vi "G4BaseTemplate_Singleton_4x4x4_ReadWriteAttribute.vi"(8 "error in (no error)":errorcluster) -> (0 "error out":errorcluster)   [LabVIEW 2016]
uses:
  <resource>/Framework/Providers/Open_GDS/ClassProviders/Provider_EndevoGOOP400/Templates/G4BaseTemplate_Singleton_4x4x4/G4BaseTemplate_Singleton_4x4x4.lvclass
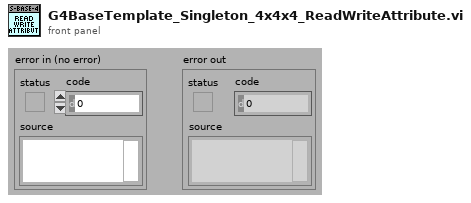
[diagram p1: front panel]
types:
  T1 = typedef "G4BaseTemplate_Singleton_4x4x4.lvclass/ObjectAttributes.ctl" = cluster{"Attribute1":dbl}
  T2 = typedef "G4BaseTemplate_Simple_4x4x4.lvclass/ObjectAttributes.ctl" = cluster{"Attribute1":dbl}
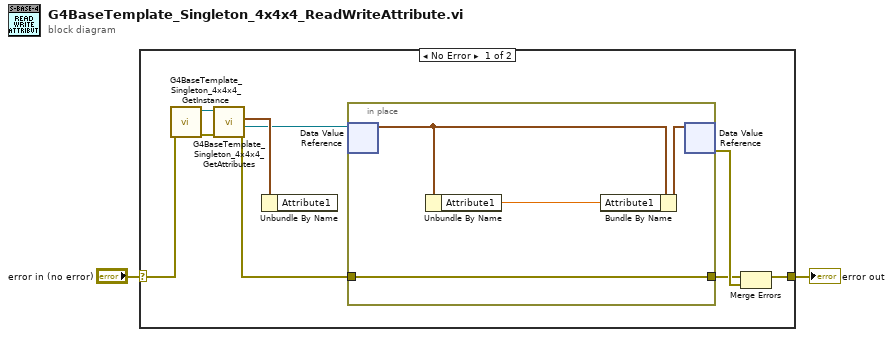
[diagram p0: block diagram]
diagram:
  n1 = case shown="No Error" "error in (no error)" {
    selector: "error in (no error)" -> [w6 w16]
    tunnel: [w9 w16] -> w1
    frame No Error {
      n2 = call <resource>:"G4BaseTemplate_Singleton_4x4x4_GetInstance.vi"("error in (no error)"=w6) -> ("error out"=w8:errorcluster, "reference out"=w7:refnum<class "G4BaseTemplate_Singleton_4x4x4.lvclass">)  [unwired: 6 in, 3 out]
      n3 = call <resource>:"G4BaseTemplate_Singleton_4x4x4_GetAttributes.vi"("error in (no error)"=w8, "reference in"=w7) -> ("error out"=w4:errorcluster, "DataRef"=w5:refnum<data-value>, "Data"=w11:T1)  [unwired: 6 in, 1 out]
      n4 = Unbundle By Name(w11) -> ()  [unwired: 1 out]
      n5 = in-place {
        in-place-border: w4 -> [w12]
        in-place-border: [w12] -> w3
        n6 = in-place-dvr #1(w5) -> (w14:T2)  [unwired: 1 out]
        n7 = Unbundle By Name(w14) -> ("Attribute1"=w13:dbl)
        n8 = Bundle By Name(cluster=w14, "Attribute1"=w13) -> (w15:T2)
        n9 = in-place-dvr #1(w15) -> (w10:errorcluster)  [unwired: 1 out]
      }
      n10 = Merge Errors(w3, w10) -> (w9:errorcluster)
    }
    frame Error {
    }
  }
  "error out" <- w1
